vi "ExtractCompletionTimesFromRankMatrix.vi"(8 "Number of  Jobs":i32=4, 9 "Number of Machines":i32=4, 10 "Processing Times":u16[][](array[numeric])=[[34, 15, 38, 95], [2, 89, 19, 7], [54, 70, 28, 34], [61, 9, 87, 29]], 11 "Rank Matrix":i32[][](array[numeric])=[[4, 1, 2, 3], [2, 3, 1, 4], [1, 4, 3, 2], [3, 2, 4, 1]]) -> (0 "Jobs On Machines":i32[][](array[numeric]), 1 "Start Times":u16[][](array[numeric]), 2 "Machine Completion Times":u16[](array[numeric]), 3 "Completion Times":u16[][](array[numeric]))   [LabVIEW 2013]
panel:
  out "output array":i32[](array[numeric])
  out "Job Completion Times":u16[](array[numeric])
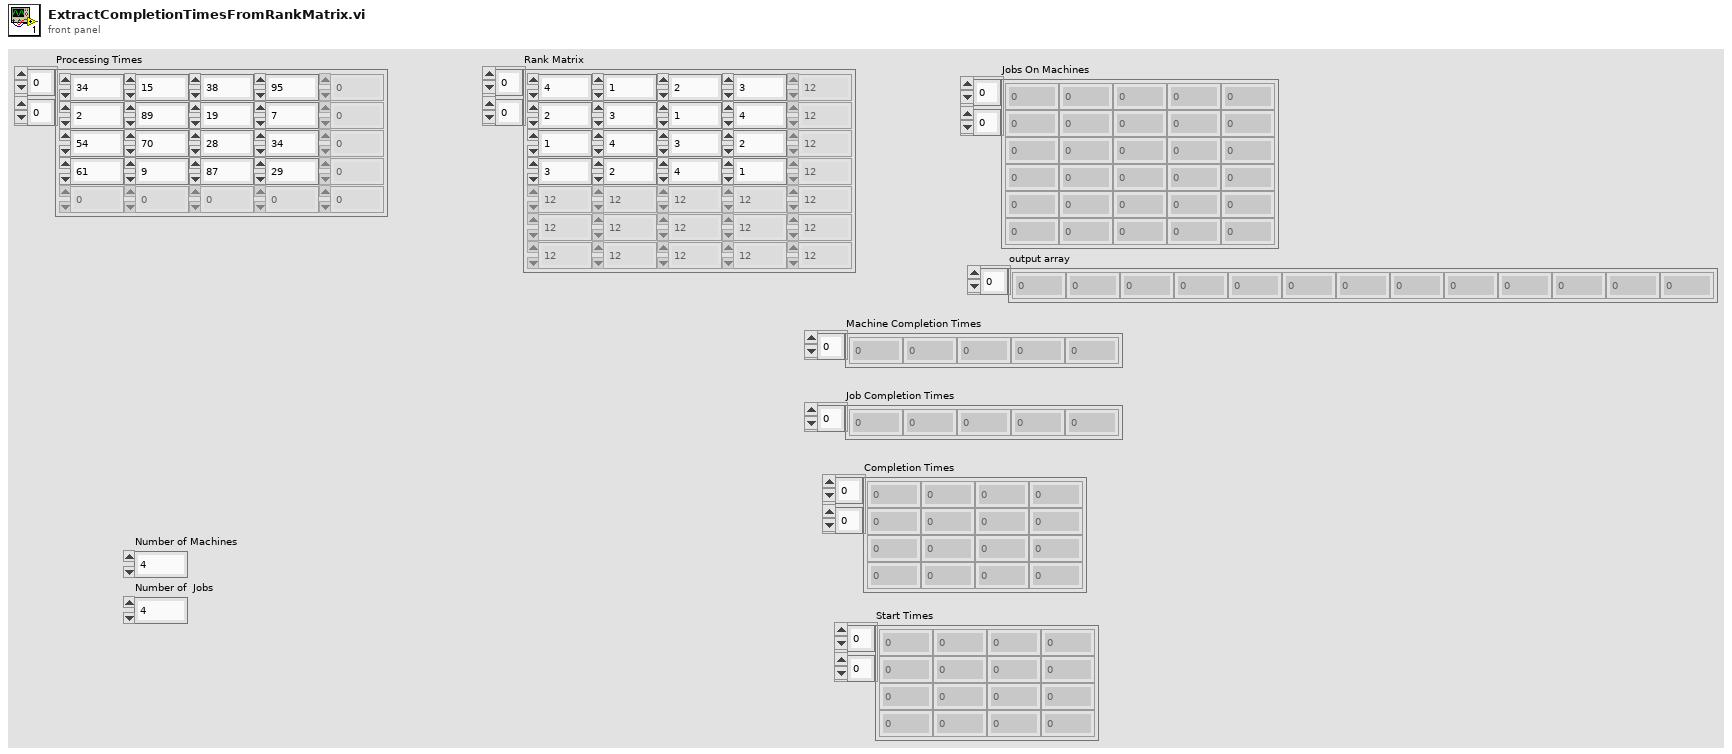
[diagram p1: front panel]
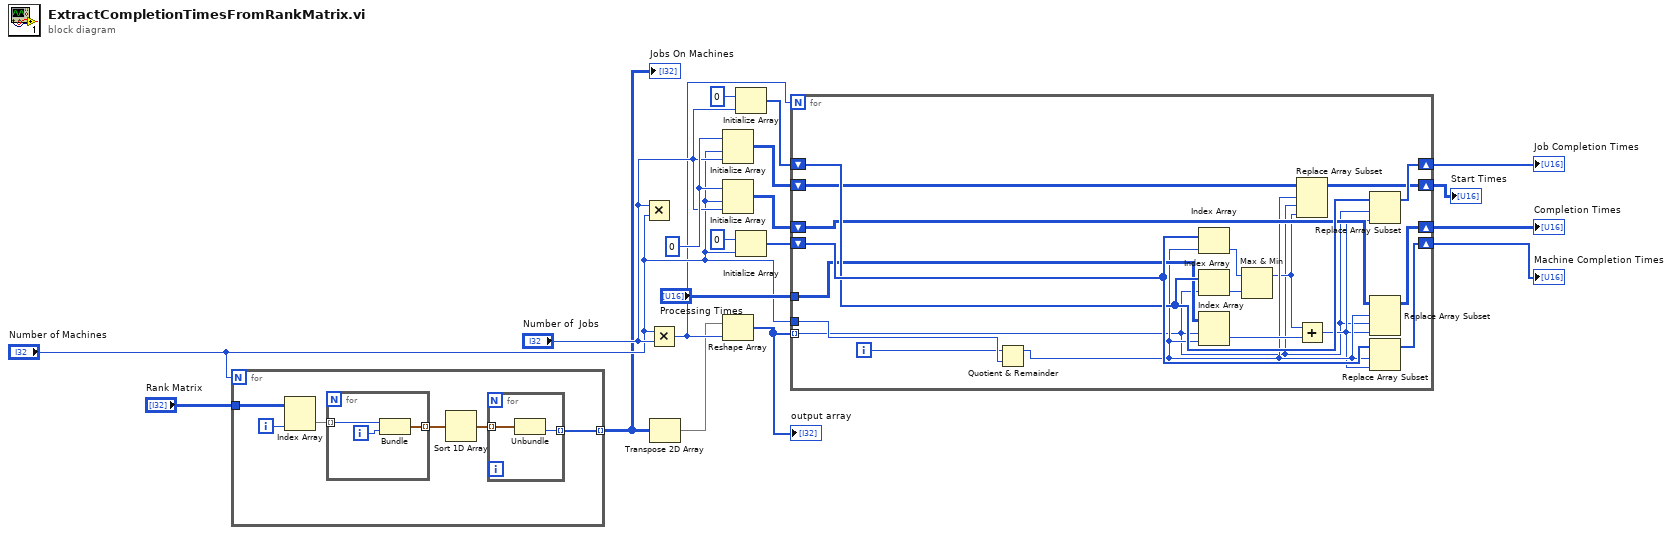
[diagram p0: block diagram]
diagram:
  w10 = u16 0 ("element")
  n1 = for {
    N: "Number of Machines" -> [_]
    tunnel: "Rank Matrix" -> [w25]
    tunnel: [w21] -> w2 mode=indexing
    i -> [w20]
    n2 = Index Array(array=w25, index (col)=w20) -> (element=w24:i32[])  [unwired: 1 in]
    n3 = for {
      tunnel: w24 -> [w30] mode=indexing
      tunnel: [w28] -> w23 mode=indexing
      i -> [w29]
      n4 = Bundle("Numeric"=w30, w29) -> (w28:cluster{"Numeric":i32, i32})  [unwired: 1 in]
    }
    n5 = Sort 1D Array(array=w23) -> (sorted array=w22:cluster{"Numeric":i32, i32}[])
    n6 = for {
      tunnel: w22 -> [w27] mode=indexing
      tunnel: [w26] -> w21 mode=indexing
      n7 = Unbundle(w27) -> (w26:i32)  [unwired: 1 out]
    }
  }
  "Jobs On Machines" <- w2
  n8 = Multiply(x="Number of  Jobs", y="Number of Machines") -> ()  [unwired: 1 out]
  n9 = Multiply(x="Number of Machines", y="Number of  Jobs") -> (x*y=w4:i32)
  n10 = Transpose 2D Array(2D array=w2) -> (transposed array=w1:i32[][])
  n11 = Initialize Array(w10, "Number of Machines", "Number of  Jobs") -> (w9:u16[][])
  n12 = Initialize Array(w10, "Number of Machines", "Number of  Jobs") -> (w14:u16[][])
  n13 = Reshape Array(w1, w4) -> (w3:i32[])
  "output array" <- w3
  n14 = Initialize Array(u16 0 ("element"), "Number of  Jobs") -> (w17:u16[])
  n15 = Initialize Array(u16 0 ("element"), "Number of Machines") -> (w16:u16[])
  n16 = for {
    N: w4 -> [_]
    shift-right: [w45] -> w12
    shift-left: w17 -> [w47]
    shift-right: [w46] -> w11
    shift-left: w16 -> [w48]
    shift-right: [w43] -> w13
    shift-left: w14 -> [w44]
    tunnel: "Processing Times" -> [w40]
    shift-right: [w41] -> w8
    shift-left: w9 -> [w42]
    tunnel: "Number of Machines" -> [w36]
    tunnel: w3 -> [w31] mode=indexing
    i -> [w35]
    n17 = Quotient & Remainder(x=w35, y=w36) -> (x-y*floor(x/y)=w34:i32)  [unwired: 1 out]
    n18 = Index Array(array=w48, index=w34) -> (element=w39:u16)
    n19 = Index Array(array=w47, index=w31) -> (element=w38:u16)
    n20 = Index Array(array=w40, index (row)=w31, index (col)=w34) -> (element=w37:u16)
    n21 = Max & Min(x=w39, y=w38) -> (max(x,y)=w33:u16)  [unwired: 1 out]
    n22 = Replace Array Subset(array=w42, new element=w33, index (row)=w34, index (col)=w31) -> (w41:u16[][])
    n23 = Add(x=w33, y=w37) -> (x+y=w32:u16)
    n24 = Replace Array Subset(array=w47, new element=w32, index=w31) -> (w45:u16[])
    n25 = Replace Array Subset(array=w44, new element=w32, index (row)=w34, index (col)=w31) -> (w43:u16[][])
    n26 = Replace Array Subset(array=w48, new element=w32, index=w34) -> (w46:u16[])
  }
  "Completion Times" <- w13
  "Job Completion Times" <- w12
  "Machine Completion Times" <- w11
  "Start Times" <- w8
